vi "Check Memory.vi"(10 "Beam":refnum<class "Beam.lvclass">, 11 "Maze In":refnum<class "Maze.lvclass">) -> (1 "key not found?":bool, 2 "Beams":refnum<class "Beam.lvclass">[](array[class]), 3 "Maze Out":refnum<class "Maze.lvclass">)   [LabVIEW 2021, in "Maze.lvclass"]
uses:
  Maze.lvclass
  Beam/Beam.lvclass
  Maze.lvclass/Maze.ctl
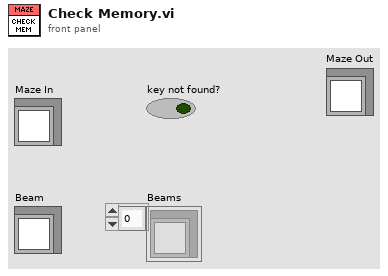
[diagram p1: front panel]
types:
  T1 = map{refnum<class "Beam.lvclass">, refnum<class "Beam.lvclass">[]}
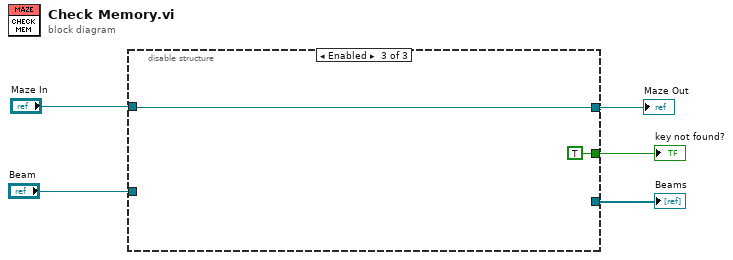
[diagram p0: block diagram]
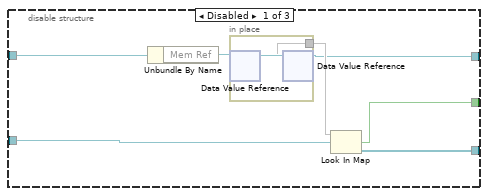
[diagram p2: hidden frame]
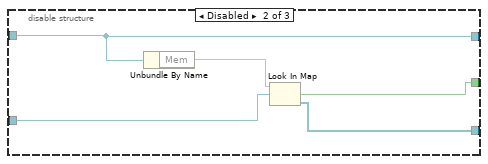
[diagram p3: hidden frame]
diagram:
  n1 = disable-structure shown="Enabled" {
    disable-tunnel: "Maze In" -> [w9 w13 w19]
    disable-tunnel: "Beam" -> [w8 w16 _]
    disable-tunnel: [w7 w15 _] -> w3
    disable-tunnel: [w6 w14 TRUE ("key not found?")] -> w2
    disable-tunnel: [w9 w13 w19] -> w1
    frame Disabled {
      n2 = Unbundle By Name(w9) -> ("Mem Ref"=w10:refnum<data-value>)
      n3 = in-place {
        in-place-border: [w12] -> w11
        n4 = in-place-dvr #1(w10) -> (w12:T1)  [unwired: 1 out]
        n5 = in-place-dvr #1() -> ()  [unwired: 1 in, 2 out]
      }
      n6 = Look In Map(map=w11, key=w8) -> (key not found?=w6:bool, value=w7:refnum<class "Beam.lvclass">[])  [unwired: 1 in]
    }
    frame Disabled {
      n7 = Unbundle By Name(w13) -> ("Mem"=w17:T1)
      n8 = Look In Map(map=w17, key=w16) -> (key not found?=w14:bool, value=w15:refnum<class "Beam.lvclass">[])  [unwired: 1 in]
    }
    frame Enabled {
    }
  }
  "Beams" <- w3
  "key not found?" <- w2
  "Maze Out" <- w1
